vi "三维图普，以及sin 重叠函数.vi"() -> ()   [LabVIEW 2023]
uses:
  <vilib>/Math Plots/3D Math Plots/3D Scatter/3D Scatter XCtrl/3D Scatter.xctl
  <vilib>/Math Plots/3D Math Plots/3D Comet/3D Comet XCtrl/3D Comet.xctl
  <vilib>/Math Plots/3D Math Plots/3D Comet/3D Comet Datatype/Public/Plot Helper (Vector).vi
  <vilib>/Utility/file.llb/Read Delimited Spreadsheet (string).vi
  <vilib>/Math Plots/3D Math Plots/3D Scatter/3D Scatter Datatype/Public/Plot Helper (Matrices).vi
  <vilib>/Math Plots/3D Math Plots/3D Scatter/3D Scatter Datatype/Public/Plot Helper (Vector).vi
  <vilib>/Math Plots/3D Math Plots/3D Scatter/3D Scatter Datatype/3D Scatter Datatype.lvclass
  <vilib>/Math Plots/3D Math Plots/3D Comet/3D Comet Datatype/3D Comet Datatype.lvclass
panel:
  out "3D Comet":refnum<class "3D Plot Datatype.lvclass">[](xcontrol)
  out "Square":dynamicdata(graph)
  out "3D Scatter 2":refnum<class "3D Plot Datatype.lvclass">[](xcontrol)
  out "XY Graph":cluster{dbl[], dbl[]}[](graph)
  out "3D Scatter":refnum<class "3D Plot Datatype.lvclass">[](xcontrol)
  # "多通道二维图练习  与 三维练习 csv"
  # "习题"
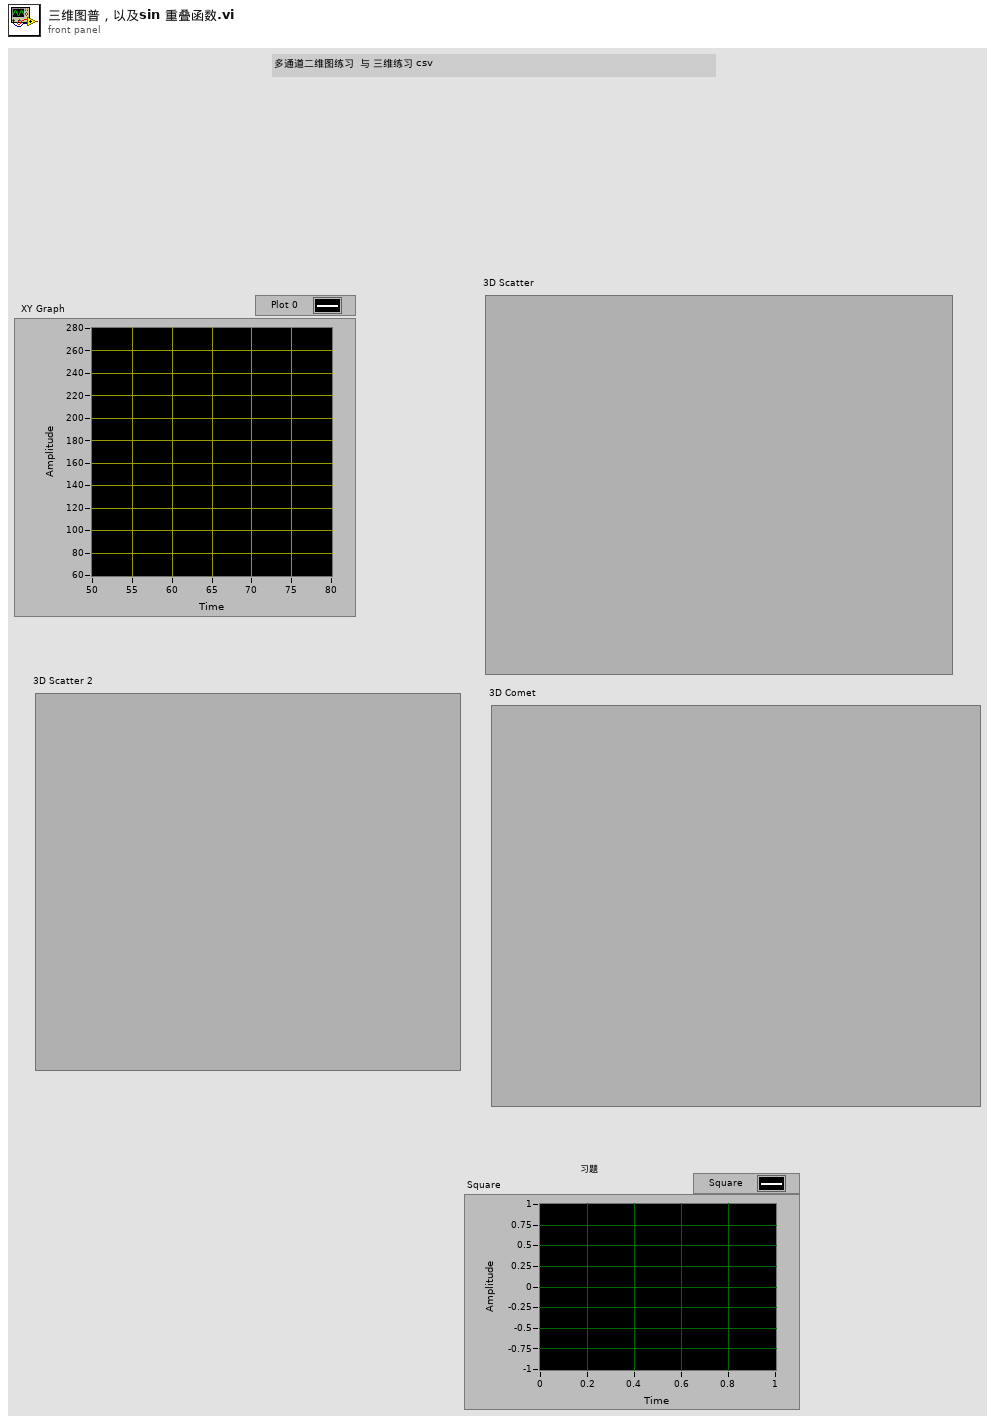
[diagram p1: front panel]
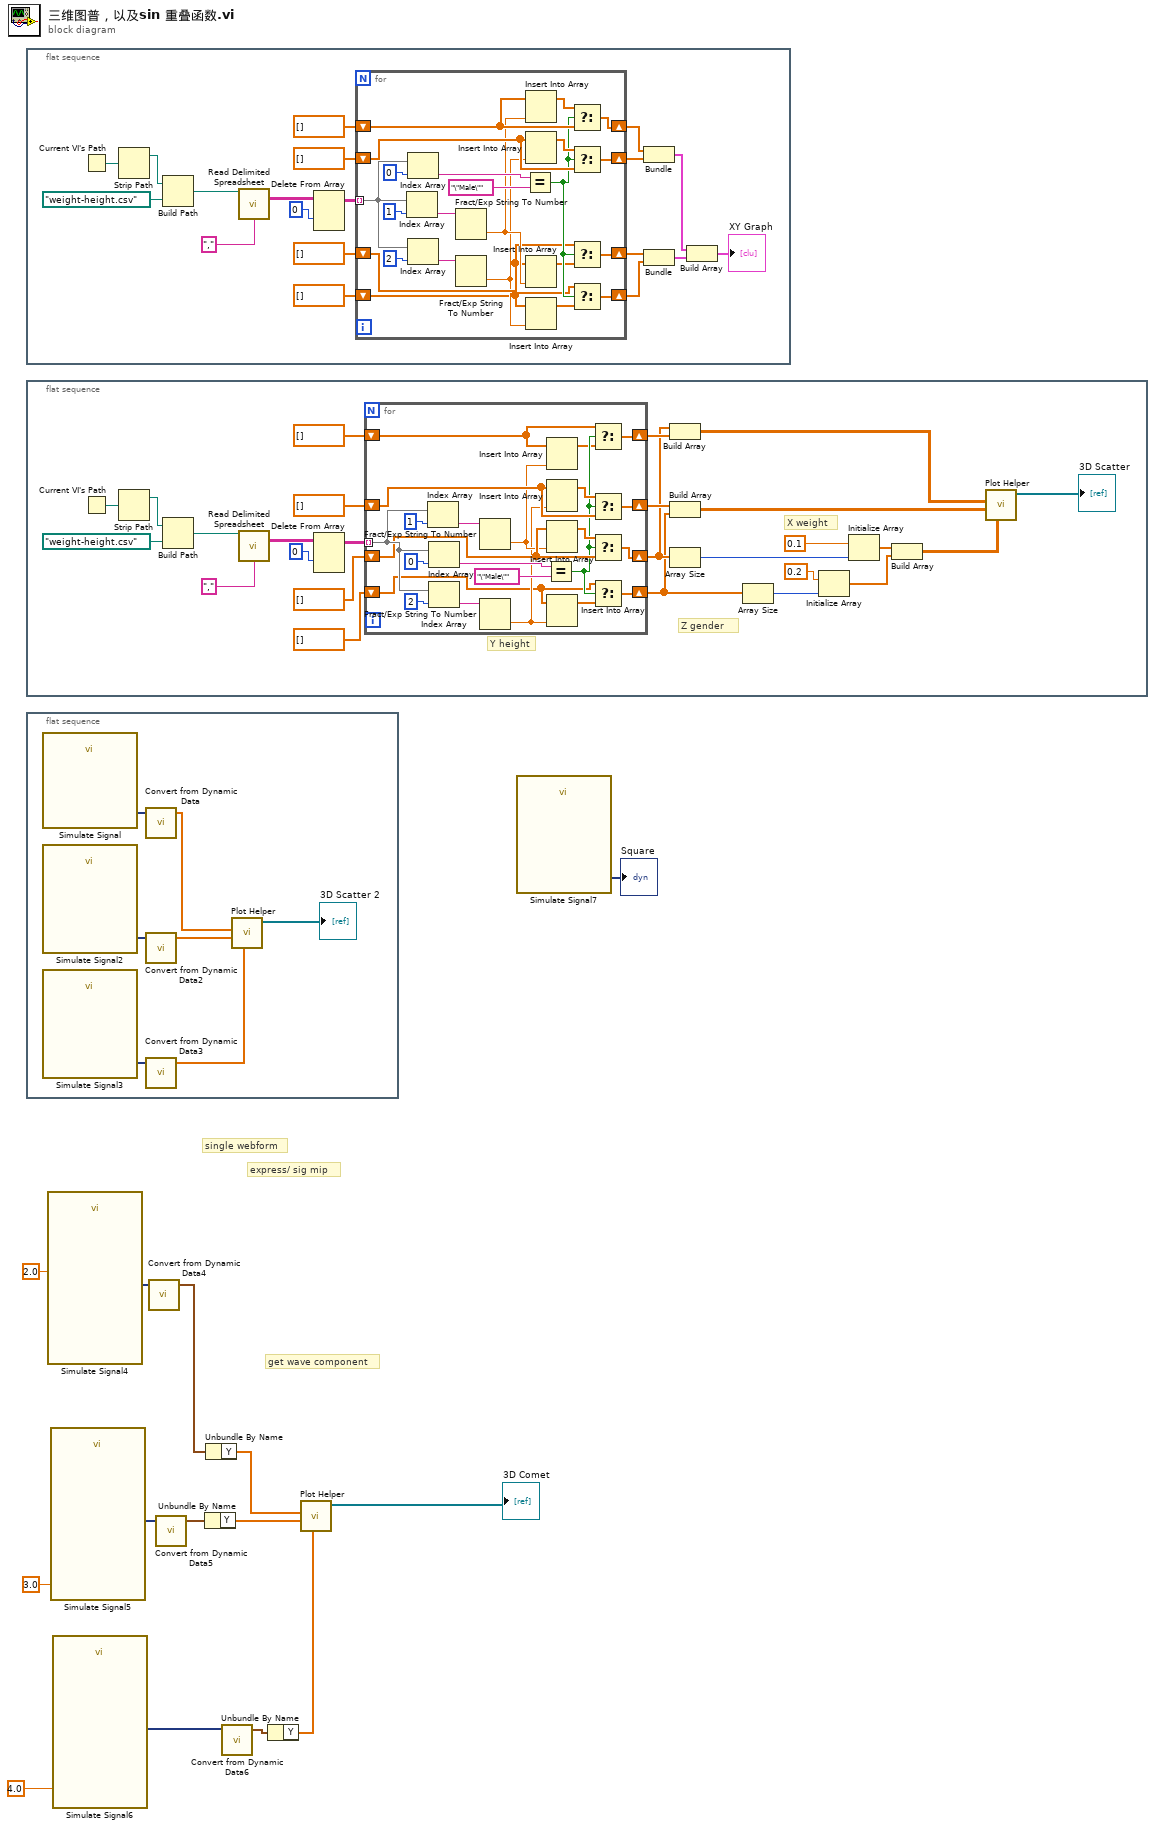
[diagram p0: block diagram]
diagram:
  # "get wave component"
  # "single webform"
  # "express/ sig mip"
  n1 = flat-sequence {
    frame #0 {
      n2 = Current VI's Path() -> (path=w33:path)
      n3 = Strip Path(path=w33) -> (stripped path=w32:path)  [unwired: 1 out]
      n4 = Build Path(base path=w32, name or relative path=path "weight-height.csv") -> (appended path=w30:path)
      n5 = call-poly <vilib>:"Read Delimited Spreadsheet.vi"("file path (dialog if empty)"=w30, "delimiter (\\t)"="," ("delimiter (\\t)")) -> ("all rows"=w28:string[][])  [unwired: 8 in, 5 out]
      n6 = Delete From Array(array=w28, index (row)=0) -> (array with subset deleted=w26:string[][])  [unwired: 2 in, 1 out]
      n7 = for {
        tunnel: w26 -> [w56] mode=indexing
        shift-right: [w47] -> w21
        shift-left: dbl[] [] -> [w46]
        shift-right: [w43] -> w20
        shift-left: dbl[] [] -> [w44]
        shift-right: [w35] -> w19
        shift-left: dbl[] [] -> [w39]
        shift-right: [w34] -> w18
        shift-left: dbl[] [] -> [w36]
        n8 = Index Array(array=w56, index=1) -> (element=w50:string)
        n9 = Index Array(array=w56, index=0) -> (element=w52:string)
        n10 = Index Array(array=w56, index=2) -> (element=w49:string)
        n11 = Fract/Exp String To Number(string=w50) -> (number=w41:dbl)  [unwired: 3 in, 1 out]
        n12 = Fract/Exp String To Number(string=w49) -> (number=w38:dbl)  [unwired: 3 in, 1 out]
        n13 = Equal?(x=w52, y="\"Male\"") -> (x = y?=w42:bool)
        n14 = Insert Into Array(array=w46, new element=w41) -> (w48:dbl[])  [unwired: 1 in]
        n15 = Insert Into Array(array=w44, new element=w38) -> (w45:dbl[])  [unwired: 1 in]
        n16 = Insert Into Array(array=w39, new element=w41) -> (w40:dbl[])  [unwired: 1 in]
        n17 = Insert Into Array(array=w36, new element=w38) -> (w37:dbl[])  [unwired: 1 in]
        n18 = Select(t=w48, s=w42, f=w46) -> (s? t:f=w47:dbl[])
        n19 = Select(t=w45, s=w42, f=w44) -> (s? t:f=w43:dbl[])
        n20 = Select(t=w39, s=w42, f=w40) -> (s? t:f=w35:dbl[])
        n21 = Select(t=w36, s=w42, f=w37) -> (s? t:f=w34:dbl[])
      }
      n22 = Bundle(w21, w20) -> (w17:cluster{dbl[], dbl[]})  [unwired: 1 in]
      n23 = Bundle(w19, w18) -> (w16:cluster{dbl[], dbl[]})  [unwired: 1 in]
      n24 = Build Array(w17, w16) -> (→"XY Graph":cluster{dbl[], dbl[]}[])
    }
  }
  n25 = flat-sequence {
    frame #0 {
      # "Z gender"
      # "Y height"
      # "X weight"
      n26 = Current VI's Path() -> (path=w82:path)
      n27 = Strip Path(path=w82) -> (stripped path=w81:path)  [unwired: 1 out]
      n28 = Build Path(base path=w81, name or relative path=path "weight-height.csv") -> (appended path=w79:path)
      n29 = call-poly <vilib>:"Read Delimited Spreadsheet.vi"("file path (dialog if empty)"=w79, "delimiter (\\t)"="," ("delimiter (\\t)")) -> ("all rows"=w77:string[][])  [unwired: 8 in, 5 out]
      n30 = Delete From Array(array=w77, index (row)=0) -> (array with subset deleted=w75:string[][])  [unwired: 2 in, 1 out]
      n31 = for {
        tunnel: w75 -> [w105] mode=indexing
        shift-right: [w96] -> w68
        shift-left: dbl[] [] -> [w95]
        shift-right: [w92] -> w69
        shift-left: dbl[] [] -> [w93]
        shift-right: [w84] -> w70
        shift-left: dbl[] [] -> [w88]
        shift-right: [w83] -> w65
        shift-left: dbl[] [] -> [w85]
        n32 = Index Array(array=w105, index=1) -> (element=w99:string)
        n33 = Index Array(array=w105, index=0) -> (element=w101:string)
        n34 = Index Array(array=w105, index=2) -> (element=w98:string)
        n35 = Fract/Exp String To Number(string=w99) -> (number=w90:dbl)  [unwired: 3 in, 1 out]
        n36 = Fract/Exp String To Number(string=w98) -> (number=w87:dbl)  [unwired: 3 in, 1 out]
        n37 = Equal?(x=w101, y="\"Male\"") -> (x = y?=w91:bool)
        n38 = Insert Into Array(array=w88, new element=w90) -> (w89:dbl[])  [unwired: 1 in]
        n39 = Insert Into Array(array=w93, new element=w87) -> (w94:dbl[])  [unwired: 1 in]
        n40 = Insert Into Array(array=w95, new element=w90) -> (w97:dbl[])  [unwired: 1 in]
        n41 = Insert Into Array(array=w85, new element=w87) -> (w86:dbl[])  [unwired: 1 in]
        n42 = Select(t=w88, s=w91, f=w89) -> (s? t:f=w84:dbl[])
        n43 = Select(t=w94, s=w91, f=w93) -> (s? t:f=w92:dbl[])
        n44 = Select(t=w97, s=w91, f=w95) -> (s? t:f=w96:dbl[])
        n45 = Select(t=w85, s=w91, f=w86) -> (s? t:f=w83:dbl[])
      }
      n46 = Build Array(w68, w70) -> (w59:dbl[][])
      n47 = Build Array(w69, w65) -> (w58:dbl[][])
      n48 = Array Size(array=w68) -> (size(s)=w67:i32)
      n49 = Array Size(array=w65) -> (size(s)=w64:i32)
      n50 = Initialize Array(0.2 ("element"), w64) -> (w61:dbl[])
      n51 = Initialize Array(0.1 ("element"), w67) -> (w62:dbl[])
      n52 = Build Array(w62, w61) -> (w57:dbl[][])
      n53 = call-poly <vilib>:"Plot Helper.vi"("z matrix"=w57, "y matrix"=w58, "x matrix"=w59) -> ("3D Plot lvclass Array out"=→"3D Scatter":refnum<class "3D Plot Datatype.lvclass">[])  [unwired: 3 in, 5 out]
    }
  }
  n54 = flat-sequence {
    frame #0 {
      n55 = call "Simulate Signal"() -> ("Sine"=w111:dynamicdata)  [unwired: 14 in, 1 out]
      n56 = call "Simulate Signal2"() -> ("Sine"=w109:dynamicdata)  [unwired: 14 in, 1 out]
      n57 = call "Simulate Signal3"() -> ("Sine"=w107:dynamicdata)  [unwired: 14 in, 1 out]
      n58 = call "Convert from Dynamic Data"("Dynamic Data Type"=w111) -> ("Array"=w110:dbl[])  [unwired: 3 in]
      n59 = call "Convert from Dynamic Data2"("Dynamic Data Type"=w109) -> ("Array"=w108:dbl[])  [unwired: 3 in]
      n60 = call "Convert from Dynamic Data3"("Dynamic Data Type"=w107) -> ("Array"=w106:dbl[])  [unwired: 3 in]
      n61 = call-poly <vilib>:"Plot Helper.vi"("z vector"=w106, "y vector"=w108, "x vector"=w110) -> ("3D Plot lvclass Array out"=→"3D Scatter 2":refnum<class "3D Plot Datatype.lvclass">[])  [unwired: 3 in, 5 out]
    }
  }
  n62 = call "Simulate Signal4"("Frequency"=2.0) -> ("Sine"=w11:dynamicdata)  [unwired: 13 in, 1 out]
  n63 = call "Simulate Signal5"("Frequency"=3.0) -> ("Sine"=w7:dynamicdata)  [unwired: 13 in, 1 out]
  n64 = call "Simulate Signal6"("Frequency"=4.0) -> ("Sine"=w6:dynamicdata)  [unwired: 13 in, 1 out]
  n65 = call "Convert from Dynamic Data4"("Dynamic Data Type"=w11) -> ("Waveform"=w10:waveform(dbl))  [unwired: 3 in]
  n66 = call "Convert from Dynamic Data5"("Dynamic Data Type"=w7) -> ("Waveform"=w9:waveform(dbl))  [unwired: 3 in]
  n67 = Unbundle By Name(w9) -> ("Y"=w3:dbl[])
  n68 = Unbundle By Name(w10) -> ("Y"=w5:dbl[])
  n69 = call "Convert from Dynamic Data6"("Dynamic Data Type"=w6) -> ("Waveform"=w8:waveform(dbl))  [unwired: 3 in]
  n70 = Unbundle By Name(w8) -> ("Y"=w4:dbl[])
  n71 = call-poly <vilib>:"Plot Helper.vi"("z vector"=w4, "y vector"=w3, "x vector"=w5) -> ("3D Plot lvclass Array out"=→"3D Comet":refnum<class "3D Plot Datatype.lvclass">[])  [unwired: 3 in, 5 out]
  n72 = call "Simulate Signal7"() -> ("Square"=→"Square":dynamicdata)  [unwired: 14 in, 1 out]
